vi "ATECC2 System Designer.vi"() -> ()   [LabVIEW 2023]
panel:
  in  "Full System Configuration":cluster{}
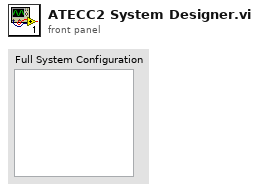
[diagram p1: front panel]
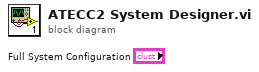
[diagram p0: block diagram]
diagram:
